vi "Build Status.vi"(8 "error in (no error)":errorcluster, 11 "Log Manager Module in":refnum<class "Log Manager Module.lvclass">) -> (0 "error out":errorcluster, 2 "Logging State":T1, 3 "Log Manager Module out":refnum<class "Log Manager Module.lvclass">)   [LabVIEW 2020, in "VolatusData.lvlib" / "Log Manager Module.lvclass"]
uses:
  Log Manager Module.lvclass
  Log Status.ctl
  Logging State.ctl
  Group State.ctl
  Logger State.ctl
  Log Manager Module.lvclass/Log Manager Module.ctl
  VolatusData.lvlib
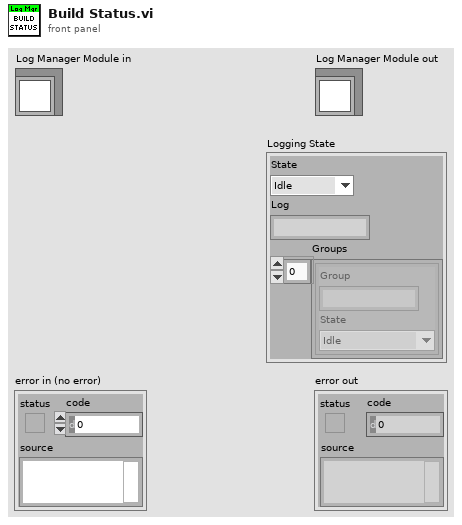
[diagram p1: front panel]
types:
  T1 = typedef "VolatusData.lvlib/Log Status.ctl" = cluster{"State":T2, "Log":string, "Groups":T3[]}
  T2 = typedef "VolatusData.lvlib/Logging State.ctl" = enum16{"Idle", "Starting", "Logging", "Stopping"}
  T3 = typedef "VolatusData.lvlib/Group State.ctl" = cluster{"Group":string, "State":T4}
  T4 = typedef "VolatusData.lvlib/Logger State.ctl" = enum16{"Unknown", "Idle", "Preparing", "Ready", "Logging", "Stopping"}
  T5 = typedef "VolatusData.lvlib/Log Manager Module.lvclass/Group Info.ctl" = cluster{"Name":string, "Loggers":map{string, T6}}
  T6 = typedef "VolatusData.lvlib/Log Manager Module.lvclass/Logger.ctl" = cluster{"ID":string, "MsgQ":refnum<class "MessageQ.lvclass">, "State":T4, "Group":string}
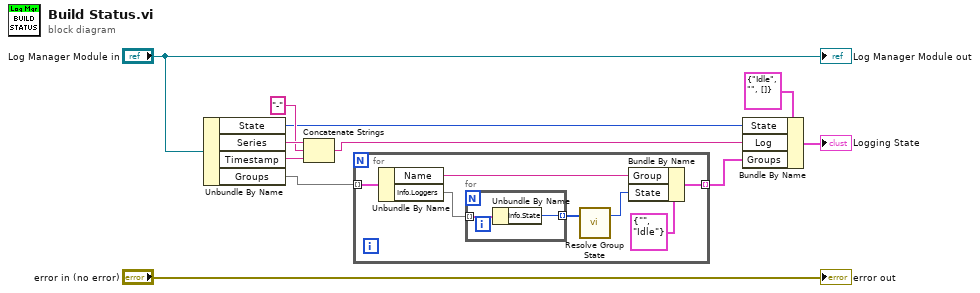
[diagram p0: block diagram]
diagram:
  n1 = Unbundle By Name("Log Manager Module in") -> ("State"=w5:T2, "Series"=w10:string, "Timestamp"=w9:string, "Groups"=w4:map{string, T5})
  n2 = Concatenate Strings(w10, "-", w9) -> (w6:string)
  n3 = for {
    tunnel: w4 -> [w18] mode=indexing
    tunnel: [w12] -> w2 mode=indexing
    n4 = Unbundle By Name(w18) -> ("Name"=w14:string, "Info.Loggers"=w17:map{string, T6})
    n5 = for {
      tunnel: w17 -> [w20] mode=indexing
      tunnel: [w19] -> w16 mode=indexing
      n6 = Unbundle By Name(w20) -> ("Info.State"=w19:T4)
    }
    n7 = call "Resolve Group State.vi"("Logger States"=w16) -> ("Group State"=w13:T4)  [unwired: 6 in]
    n8 = Bundle By Name(cluster=T3 {"Group"="", "State"=enum."Idle"} ("Group State"), "Group"=w14, "State"=w13) -> (w12:T3)
  }
  n9 = Bundle By Name(cluster=T1 {"State"=enum."Idle", "Log"="", "Groups"=[]} ("Log Status"), "State"=w5, "Log"=w6, "Groups"=w2) -> (→"Logging State":T1)
  "error out" <- "error in (no error)"
  "Log Manager Module out" <- "Log Manager Module in"
